vi "mark_volume.vi"(10 "element":T1=255, 11 "marksArray":T3[](array[typedef])) -> (3 "volume":T2)   [LabVIEW 2015, in "PolyVIEW.lvclass"]
uses:
  PolyVIEW.lvclass
  actors/world/typedefs/markValue_cluster.ctl
  actors/world/typedefs/markValue.ctl
  actors/world/typedefs/markVolume.ctl
  actors/world/world.lvlib
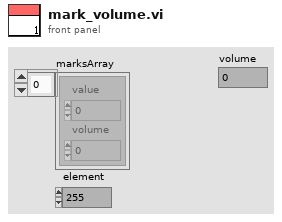
[diagram p1: front panel]
types:
  T1 = typedef "world.lvlib/markValue.ctl" = u8
  T2 = typedef "world.lvlib/markVolume.ctl" = u16
  T3 = typedef "world.lvlib/markValue_cluster.ctl" = cluster{"value":T1, "volume":T2}
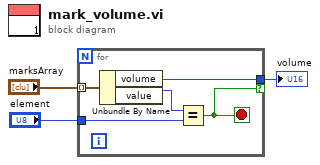
[diagram p0: block diagram]
diagram:
  n1 = for {
    tunnel: "marksArray" -> [w8] mode=indexing
    tunnel: [w7] -> w2 if=w4
    tunnel: "element" -> [w5]
    stop <- w4 stop-if-true
    n2 = Unbundle By Name(w8) -> ("volume"=w7:T2, "value"=w6:T1)
    n3 = Equal?(x=w6, y=w5) -> (x = y?=w4:bool)
  }
  "volume" <- w2
